vi "mapClassNameToNodeEnum.vi"(8 "error in (no error)":errorcluster, 10 "Class Name":string, 11 "Project in":refnum<class "Project.lvclass">) -> (0 "error out":errorcluster, 2 "NodeSelection":T1, 3 "Project out":refnum<class "Project.lvclass">)   [LabVIEW 2016, in "Project.lvclass"]
uses:
  Project.lvclass
  Typedefs/NodeSelection.ctl
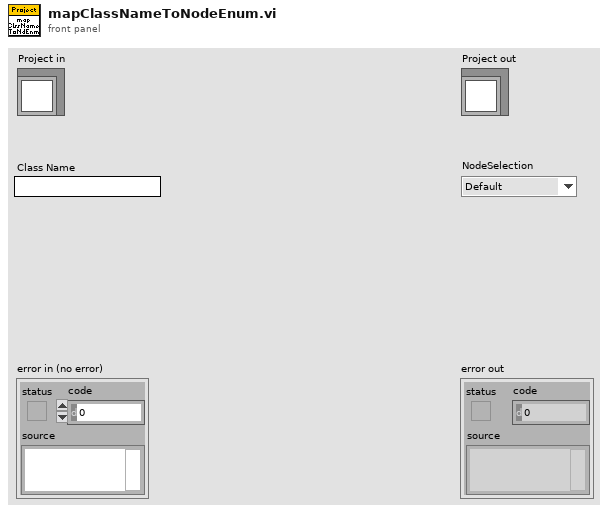
[diagram p1: front panel]
types:
  T1 = typedef "NodeSelection.ctl" = enum16{"Default", "CaseStructure", "EventStructure", "FlatSequence", "ForLoop", "WhileLoop"}
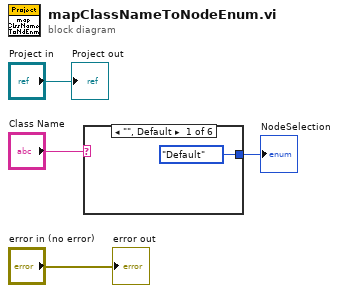
[diagram p0: block diagram]
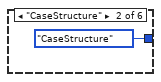
[diagram p2: hidden frame]
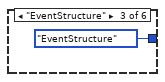
[diagram p3: hidden frame]
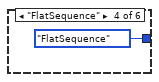
[diagram p4: hidden frame]
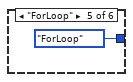
[diagram p5: hidden frame]
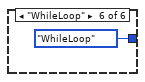
[diagram p6: hidden frame]
diagram:
  n1 = case shown="\"\", Default" "Class Name" {
    tunnel: [NodeSelection."Default" ("NodeSelection") NodeSelection."CaseStructure" ("NodeSelection") NodeSelection."EventStructure" ("NodeSelection") NodeSelection."FlatSequence" ("NodeSelection") NodeSelection."ForLoop" ("NodeSelection") NodeSelection."WhileLoop" ("NodeSelection")] -> w1
    frame "", Default {
    }
    frame "CaseStructure" {
    }
    frame "EventStructure" {
    }
    frame "FlatSequence" {
    }
    frame "ForLoop" {
    }
    frame "WhileLoop" {
    }
  }
  "NodeSelection" <- w1
  "error out" <- "error in (no error)"
  "Project out" <- "Project in"
